vi "Get Measurement Details.vi"(8 "error in":errorcluster, 11 "MeasurementPluginService in":refnum<class "MeasurementPluginService.lvclass">) -> (0 "error out":errorcluster, 1 "Service Class":string, 2 "Measurement Details":T2, 3 "MeasurementPluginService out":refnum<class "MeasurementPluginService.lvclass">, 4 "Measurement Annotations":T1)   [LabVIEW 2020, in "MeasurementLink Measurement Server.lvlib" / "MeasurementPluginService.lvclass"]
uses:
  MeasurementPluginService.lvclass
  Helpers/TypeDefs/MeasurementDetails.ctl
  Helpers/TypeDefs/MeasurementAnnotations.ctl
  MeasurementLink Measurement Server.lvlib
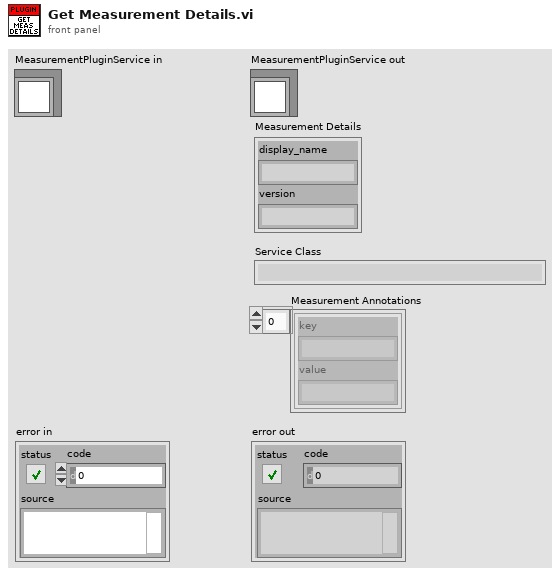
[diagram p1: front panel]
types:
  T1 = typedef "MeasurementLink Measurement Server.lvlib/MeasurementAnnotations.ctl" = cluster{"key":string, "value":string}[]
  T2 = typedef "MeasurementLink Measurement Server.lvlib/MeasurementDetails.ctl" = cluster{"display_name":string, "version":string}
  T3 = typedef "MeasurementLink Measurement Server.lvlib/MeasurementPluginService.lvclass/Plugin Paths.ctl" = cluster{"Get Measurement Details VI Path":path, "Get Type Specializations VI Path":path, "Get UI Details VI Path":path, "Measurement Logic VI Path":path, "Measurement Configuration CTL Path":path, "Measurement Results CTL Path":path}
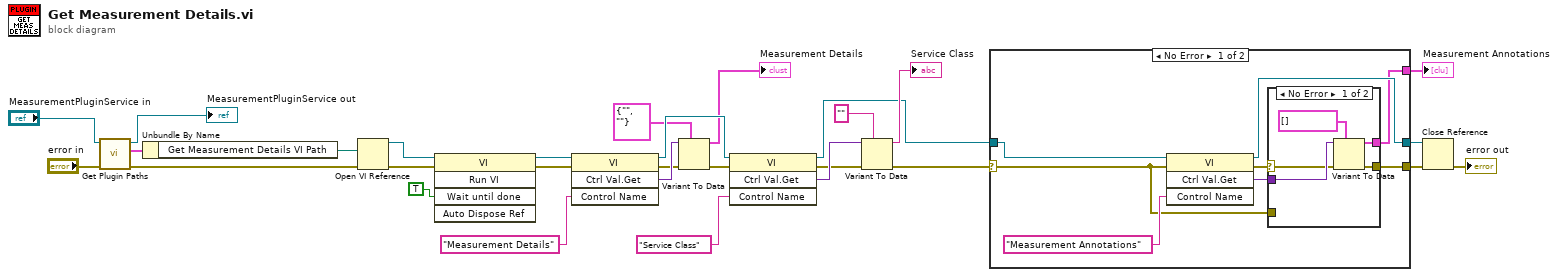
[diagram p0: block diagram]
diagram:
  n1 = call-dynamic "Get Plugin Paths.vi"("error in (no error)"="error in", "MeasurementPluginService in"="MeasurementPluginService in") -> ("error out"=w9:errorcluster, "Plugin Paths"=w26:T3, "MeasurementPluginService out"=→"MeasurementPluginService out":refnum<class "MeasurementPluginService.lvclass">)  [unwired: 7 in]
  n2 = Unbundle By Name(w26) -> ("Get Measurement Details VI Path"=w11:path)
  n3 = Open VI Reference(vi path=w11, error in (no error)=w9) -> (vi reference=w25:refnum<vi>, error out=w18:errorcluster)  [unwired: 4 in]
  n4 = invoke class="VI" method="Run VI"(reference=w25, error in=w18, "Wait until done"=TRUE ("Wait Until Done")) -> (reference out=w23:refnum<vi>, error out=w19:errorcluster)  [unwired: 2 in, 3 out]
  n5 = invoke class="VI" method="Ctrl Val.Get"(reference=w23, error in=w19, "Control Name"="Measurement Details") -> (reference out=w20:refnum<vi>, error out=w16:errorcluster, "Get Control Value Variant"=w17:variant)  [unwired: 1 in, 1 out]
  n6 = Variant To Data(error in=w16, type=T2 {"display_name"="", "version"=""} ("MeasurementDetails"), Variant=w17) -> (data=→"Measurement Details":T2, error out=w15:errorcluster)
  n7 = invoke class="VI" method="Ctrl Val.Get"(reference=w20, error in=w15, "Control Name"="Service Class") -> (reference out=w4:refnum<vi>, error out=w13:errorcluster, "Get Control Value Variant"=w14:variant)  [unwired: 1 in, 1 out]
  n8 = Variant To Data(error in=w13, type="", Variant=w14) -> (data=→"Service Class":string, error out=w1:errorcluster)
  n9 = case shown="No Error" w1 {
    selector: w1 -> [w30 w45]
    tunnel: [w37 w45] -> w5
    tunnel: w4 -> [w36 w44]
    tunnel: [w35 w44] -> w3
    tunnel: [w32 _] -> w2
    frame No Error {
      n10 = invoke class="VI" method="Ctrl Val.Get"(reference=w36, error in=w30, "Control Name"="Measurement Annotations") -> (reference out=w35:refnum<vi>, error out=w31:errorcluster, "Get Control Value Variant"=w34:variant)  [unwired: 1 in, 1 out]
      n11 = case shown="No Error" w31 {
        selector: w31 -> [w38 _]
        tunnel: [w42 w43] -> w37
        tunnel: w34 -> [w41 _]
        tunnel: [w39 _] -> w32
        tunnel: w30 -> [_ w43]
        frame No Error {
          n12 = Variant To Data(error in=w38, type=T1 [] ("MeasurementAnnotations"), Variant=w41) -> (data=w39:T1, error out=w42:errorcluster)
        }
        frame Error {
        }
      }
    }
    frame Error {
    }
  }
  "Measurement Annotations" <- w2
  n13 = Close Reference(reference=w3, error in (no error)=w5) -> (error out=→"error out":errorcluster)
